vi "G#Object_Create.vi"(0 "reference in":refnum<class "G#Interface.lvclass">, 3 "control values":variant[](array[variant]), 5 "error in (no error)":errorcluster) -> (14 "reference out":refnum<class "G#Interface.lvclass">, 19 "error out":errorcluster)   [LabVIEW 2017, in "G#Interface.lvclass"]
doc: "The G#Interface default constructor. The first element in the array must be the path to the implementing class or a G#object to the implementing object. Remaining elements are passed as arguments to the default constructor of the implementing class."
uses:
  <vilib>/addons/_AddQ/G#Interface/G#Interface.lvclass
  <vilib>/addons/_AddQ/G#Object/G#Object.lvclass
panel:
  # "The first element in the array must be the path to the\nimplementing class or a G#object to the implementing object.\nRemaining elements are passed as arguments to the\ndefault constructor of the implementing class."
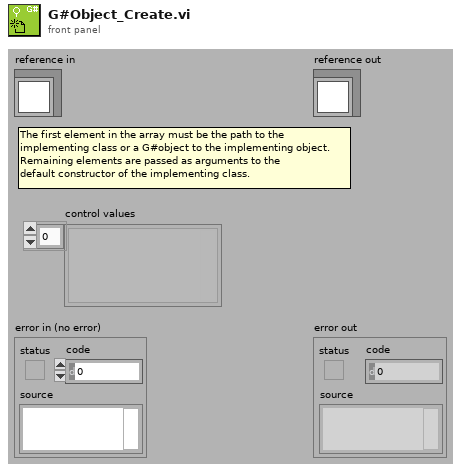
[diagram p1: front panel]
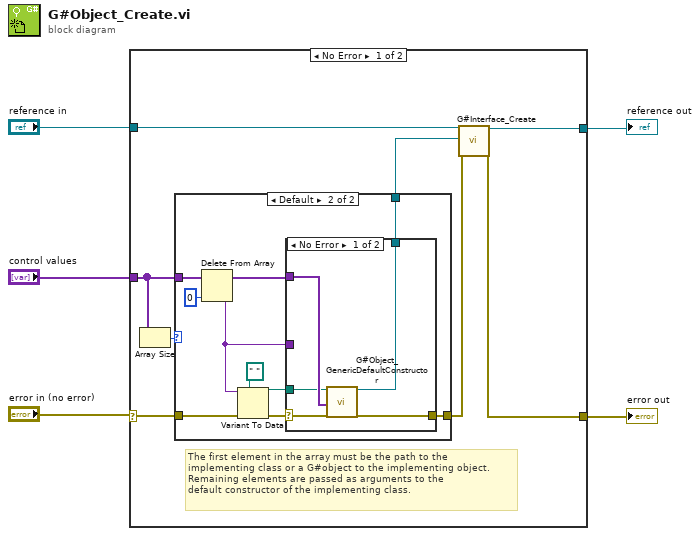
[diagram p0: block diagram]
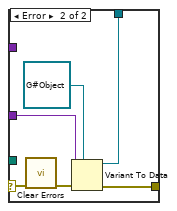
[diagram p3: hidden frame]
diagram:
  n1 = case shown="No Error" "error in (no error)" {
    selector: "error in (no error)" -> [w13 w37]
    tunnel: [w9 w37] -> w4
    tunnel: "reference in" -> [w12 w36]
    tunnel: "control values" -> [w7 _]
    tunnel: [w8 w36] -> w1
    frame No Error {
      # "The first element in the array must be the path to the\nimplementing class or a G#object to the implementing object.\nRemaining elements are passed as arguments to the\ndefault constructor of the implementing class."
      n2 = Array Size(array=w7) -> (size(s)=w6:i32)
      n3 = case shown="Default" w6 {
        tunnel: w13 -> [w14 w23]
        tunnel: [_ w19] -> w11
        tunnel: [w14 w18] -> w10
        tunnel: w7 -> [_ w17]
        frame 0 {
        }
        frame Default {
          n4 = Delete From Array(array=w17, index=0) -> (deleted portion=w15:variant, array with subset deleted=w22:variant[])  [unwired: 1 in]
          n5 = Variant To Data(error in=w23, type=path " ", Variant=w15) -> (data=w20:path, error out=w16:errorcluster)
          n6 = case shown="No Error" w16 {
            selector: w16 -> [w25 w31]
            tunnel: w22 -> [w29 _]
            tunnel: w20 -> [w28 _]
            tunnel: [w27 w32] -> w19
            tunnel: [w26 w33] -> w18
            tunnel: w15 -> [_ w35]
            frame No Error {
              n7 = call <vilib>:"G#Object_GenericDefaultConstructor.vi"("class path"=w28, "control values"=w29, "error in (no error)"=w25) -> ("reference out"=w27:refnum<class "G#Object.lvclass">, "error out"=w26:errorcluster)  [unwired: 14 in, 1 out]
            }
            frame Error {
              n8 = call <vilib>:"Clear Errors.vi"("error in (no error)"=w31) -> ("error out"=w30:errorcluster)  [unwired: 5 in, 1 out]
              n9 = Variant To Data(error in=w30, type=refnum<class "G#Object.lvclass"> refnum ("G#Object in"), Variant=w35) -> (data=w32:refnum<class "G#Object.lvclass">, error out=w33:errorcluster)
            }
          }
        }
      }
      n10 = call-dynamic "G#Interface_Create.vi"("reference in"=w12, "G#Object in"=w11, "error in (no error)"=w10) -> ("reference out"=w8:refnum<class "G#Interface.lvclass">, "error out"=w9:errorcluster)  [unwired: 15 in]
    }
    frame Error {
    }
  }
  "error out" <- w4
  "reference out" <- w1
